vi "AI IRQ UpdateState.vi"(0 "XRef":T15, 1 "Old State":T6, 2 "Version":T13) -> (14 "Is Good?":T9, 15 "Reply":T12, 16 "Fatal Error Out":T11, 17 "State Out":T1)   [LabVIEW 2021, in "myRIO Register AI IRQ.xnode"]
uses:
  <vilib>/myRIO/Instrument Drivers/IRQ/IO IRQ/vis/myRIO Register AI IRQ.xnode
  <vilib>/XNodeSupport/XNodeXNodeRef.ctl
  <vilib>/XNodeSupport/XNodeVariant.ctl
  <vilib>/XNodeSupport/XNodeVersion.ctl
  <vilib>/XNodeSupport/XNodeUShort.ctl
  <vilib>/XNodeSupport/XNodeBool.ctl
  <vilib>/XNodeSupport/XNodeStringArray.ctl
  <vilib>/XNodeSupport/XNodeString.ctl
  <vilib>/XNodeSupport/XNodeErrorCluster.ctl
  <vilib>/myRIO/Instrument Drivers/IRQ/IO IRQ/vis/AI IRQ State.ctl
  <vilib>/myRIO/Common/Instrument Driver Framework/Utilities/typedefs/myRIOXPeripheral.ctl
  <vilib>/XNodeSupport/XNodeTerm4Array.ctl
  <vilib>/XNodeSupport/XNodeTerm4.ctl
  <vilib>/XNodeSupport/XNodeRect32.ctl
  <vilib>/XNodeSupport/XNodeInt.ctl
  <vilib>/XNodeSupport/XNodeTermDirection.ctl
  <vilib>/XNodeSupport/NI_XNodeSupport.lvlib
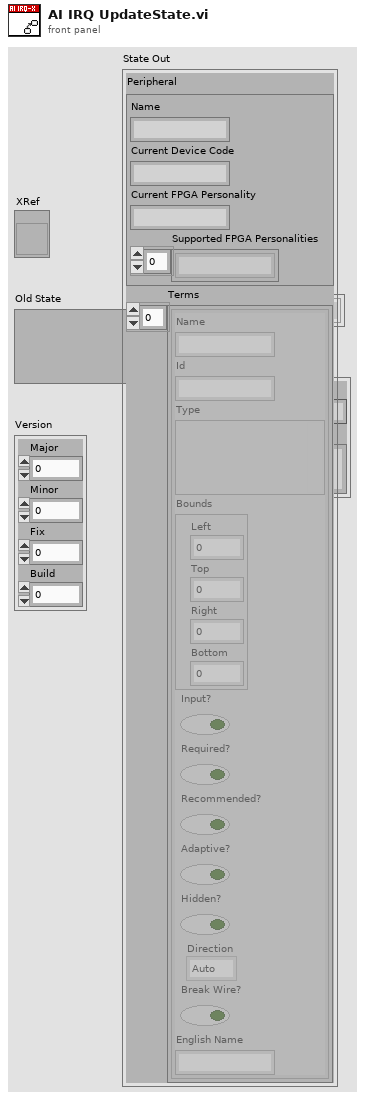
[diagram p1: front panel]
types:
  T1 = typedef "myRIO Register AI IRQ.xnode/AI IRQ State.ctl" = cluster{"Peripheral":T2, "Terms":T3}
  T2 = typedef "myRIOXPeripheral.ctl" = cluster{"Name":string, "Current Device Code":string, "Current FPGA Personality":string, "Supported FPGA Personalities":string[]}
  T3 = typedef "NI_XNodeSupport.lvlib/XNodeTerm4Array.ctl" = T4[]
  T4 = typedef "NI_XNodeSupport.lvlib/XNodeTerm4.ctl" = cluster{"Name":T5, "Id":T5, "Type":T6, "Bounds":T7, "Input?":T9, "Required?":T9, "Recommended?":T9, "Adaptive?":T9, "Hidden?":T9, "Direction":T10, "Break Wire?":T9, "English Name":T5}
  T5 = typedef "NI_XNodeSupport.lvlib/XNodeString.ctl" = string
  T6 = typedef "NI_XNodeSupport.lvlib/XNodeVariant.ctl" = variant
  T7 = typedef "NI_XNodeSupport.lvlib/XNodeRect32.ctl" = cluster{"Left":T8, "Top":T8, "Right":T8, "Bottom":T8}
  T8 = typedef "NI_XNodeSupport.lvlib/XNodeInt.ctl" = i32
  T9 = typedef "NI_XNodeSupport.lvlib/XNodeBool.ctl" = bool
  T10 = typedef "NI_XNodeSupport.lvlib/XNodeTermDirection.ctl" = enum32{"Auto", "Up", "Down", "Left", "Right", "Center"}
  T11 = typedef "NI_XNodeSupport.lvlib/XNodeErrorCluster.ctl" = errorcluster
  T12 = typedef "NI_XNodeSupport.lvlib/XNodeStringArray.ctl" = T5[]
  T13 = typedef "NI_XNodeSupport.lvlib/XNodeVersion.ctl" = cluster{"Major":T14, "Minor":T14, "Fix":T14, "Build":T14}
  T14 = typedef "NI_XNodeSupport.lvlib/XNodeUShort.ctl" = u16
  T15 = typedef "NI_XNodeSupport.lvlib/XNodeXNodeRef.ctl" = refnum<vi>
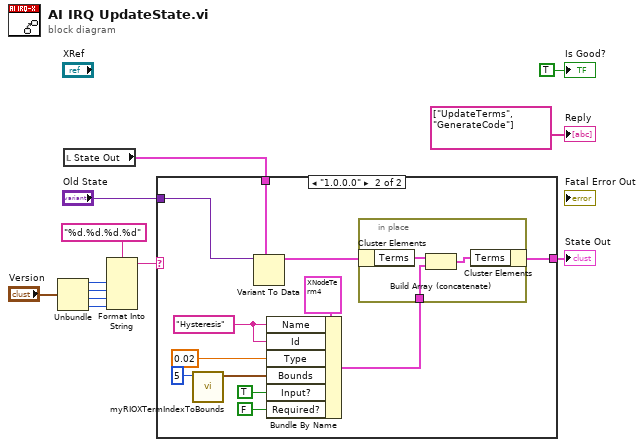
[diagram p0: block diagram]
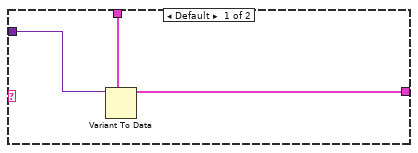
[diagram p2: hidden frame]
diagram:
  n1 = Unbundle("Version") -> ("Major"=w6:T14, "Minor"=w7:T14, "Fix"=w8:T14, "Build"=w9:T14)
  n2 = local read "State Out"() -> (w1:T1)
  n3 = Format Into String(format string="%d.%d.%d.%d", w6, w7, w8, w9) -> (resulting string=w4:string)  [unwired: 2 in, 1 out]
  n4 = case shown="\"1.0.0.0\"" w4 {
    tunnel: "Old State" -> [w15 w26]
    tunnel: [w14 w24] -> w2
    tunnel: w1 -> [w13 w27]
    frame Default {
      n5 = Variant To Data(type=w13, Variant=w15) -> (data=w14:T1)  [unwired: 1 in, 1 out]
    }
    frame "1.0.0.0" {
      w21 = T5 "Hysteresis" ("Name")
      n6 = call <vilib>:"myRIOXTermIndexToBounds.vi"("Index"=5) -> ("Bounds"=w19:T7)  [unwired: 10 in]
      n7 = Variant To Data(type=w27, Variant=w26) -> (data=w25:T1)  [unwired: 1 in, 1 out]
      n8 = Bundle By Name(cluster=T4 {"Name"="", "Id"="", "Type"=variant, "Bounds"={"Left"=0, "Top"=0, "Right"=0, "Bottom"=0}, "Input?"=FALSE, "Required?"=FALSE, "Recommended?"=FALSE, "Adaptive?"=FALSE, "Hidden?"=FALSE, "Direction"=enum."Auto", "Break Wire?"=FALSE, "English Name"=""} ("Error In Term Constant"), "Name"=w21, "Id"=w21, "Type"=0.02 ("Threshold"), "Bounds"=w19, "Input?"=T9 TRUE, "Required?"=T9 FALSE) -> (w16:T4)
      n9 = in-place {
        in-place-border: w16 -> [w28]
        n10 = in-place-cluster #1(w25) -> ("Terms"=w30:T3)
        n11 = Build Array (concatenate)(w30, w28) -> (w29:T3)
        n12 = in-place-cluster #1("Terms"=w29) -> (w24:T1)
      }
    }
  }
  "State Out" <- w2
  "Is Good?" <- T9 TRUE ("Is Good?")
  "Reply" <- T12 ["UpdateTerms", "GenerateCode"] ("Reply")
